vi "analise-motor.vi"() -> ()   [LabVIEW 2014]
panel:
  out "Waveform Graph":dbl[](graph)
  out "size(s)":i32
  out "subarray":dbl[](array[numeric]) format="%_20g"
  in  "Waveform Graph 2":dbl[][](graph)=[[0.0, 0.0, 1.0, 1.0, 1.0, 1.0, 1.0, 1.0, 1.0, 1.0, 1.0, 1.0, 1.0, 1.0, 1.0, 1.0, 1.0, 1.0, 1.0, 1.0, 1.0, 1.0, 1.0, 1.0, 1.0, 1.0, 1.0, 1.0, 1.0, 1.0, 1.0, 1.0, 1.0, 1.0, 1.0, 1.0, 1.0, 1.0, 1.0, 1.0, 1.0, 1.0, 1.0, 1.0, 1.0, 1.0, 1.0, 1.0, 1.0, 1.0, 1.0, 1.0, 1.0, 1.0, 1.0, 1.0, 1.0, 1.0, 1.0, 1.0, 1.0, 1.0, 1.0, 1.0, 1.0, 1.0, 1.0, 1.0, 1.0, 1.0, 1.0, 1.0, 1.0, 0.0, 0.0, 0.0, 0.0, 0.0, 0.0, 0.0, 0.0, 0.0, 0.0, 0.0, 0.0, 0.0, 0.0, 0.0, 0.0, 0.0, 0.0, 0.0, 0.0, 0.0, 0.0, 0.0, 0.0, 0.0, 0.0, 0.0, 0.0, 0.0, 0.0, 0.0, 0.0, 0.0, 0.0, 0.0, 0.0, 0.0], [0.0, 0.0, 0.0, 0.011164878731343308, 0.011164878731343308, 0.011164878731343308, 0.011164878731343308, 0.011164878731343308, 0.10415694962686572, 0.10415694962686572, 0.10415694962686572, 0.10415694962686572, 0.29133628731343275, 0.29133628731343275, 0.29133628731343275, 0.29133628731343275, 0.29133628731343275, 0.5729652518656717, 0.5729652518656717, 0.5729652518656717, 0.5729652518656717, 0.947440531716418, 0.947440531716418, 0.947440531716418, 0.947440531716418, 0.947440531716418, 1.4163654384328357, 1.4163654384328357, 1.4163654384328357, 1.4163654384328357, 1.4163654384328357, 1.9599755130597014, 1.9599755130597014, 1.9599755130597014, 1.9599755130597014, 1.9599755130597014, 2.5121560167910446, 2.5121560167910446, 2.5121560167910446, 2.5121560167910446, 3.0620044309701493, 3.0620044309701493, 3.0620044309701493, 3.0620044309701493, 3.0620044309701493, 3.604390158582089, 3.604390158582089, 3.604390158582089, 3.604390158582089, 3.604390158582089, 4.070195895522388, 4.070195895522388, 4.070195895522388, 4.070195895522388, 4.440794076492537, 4.440794076492537, 4.440794076492537, 4.440794076492537, 4.440794076492537, 4.717788013059701, 4.717788013059701, 4.717788013059701, 4.717788013059701, 4.717788013059701, 4.901294309701492, 4.901294309701492, 4.901294309701492, 4.901294309701492, 4.901294309701492, 4.99052588619403, 4.99052588619403, 4.99052588619403, 4.99052588619403, 5.000145755597015, 5.000145755597015, 5.000145755597015, 5.000145755597015, 5.000145755597015, 5.000029151119403, 5.000029151119403, 5.000029151119403, 5.000029151119403, 5.000029151119403, 5.0, 5.0, 5.0, 5.0, 5.0, 5.0, 5.0, 5.0, 5.0, 5.0, 5.0, 5.0, 5.0, 5.0, 5.0, 5.0, 5.0, 5.0, 5.0, 5.0, 5.0, 5.0, 5.0, 5.0, 5.0, 5.0, 5.0]]
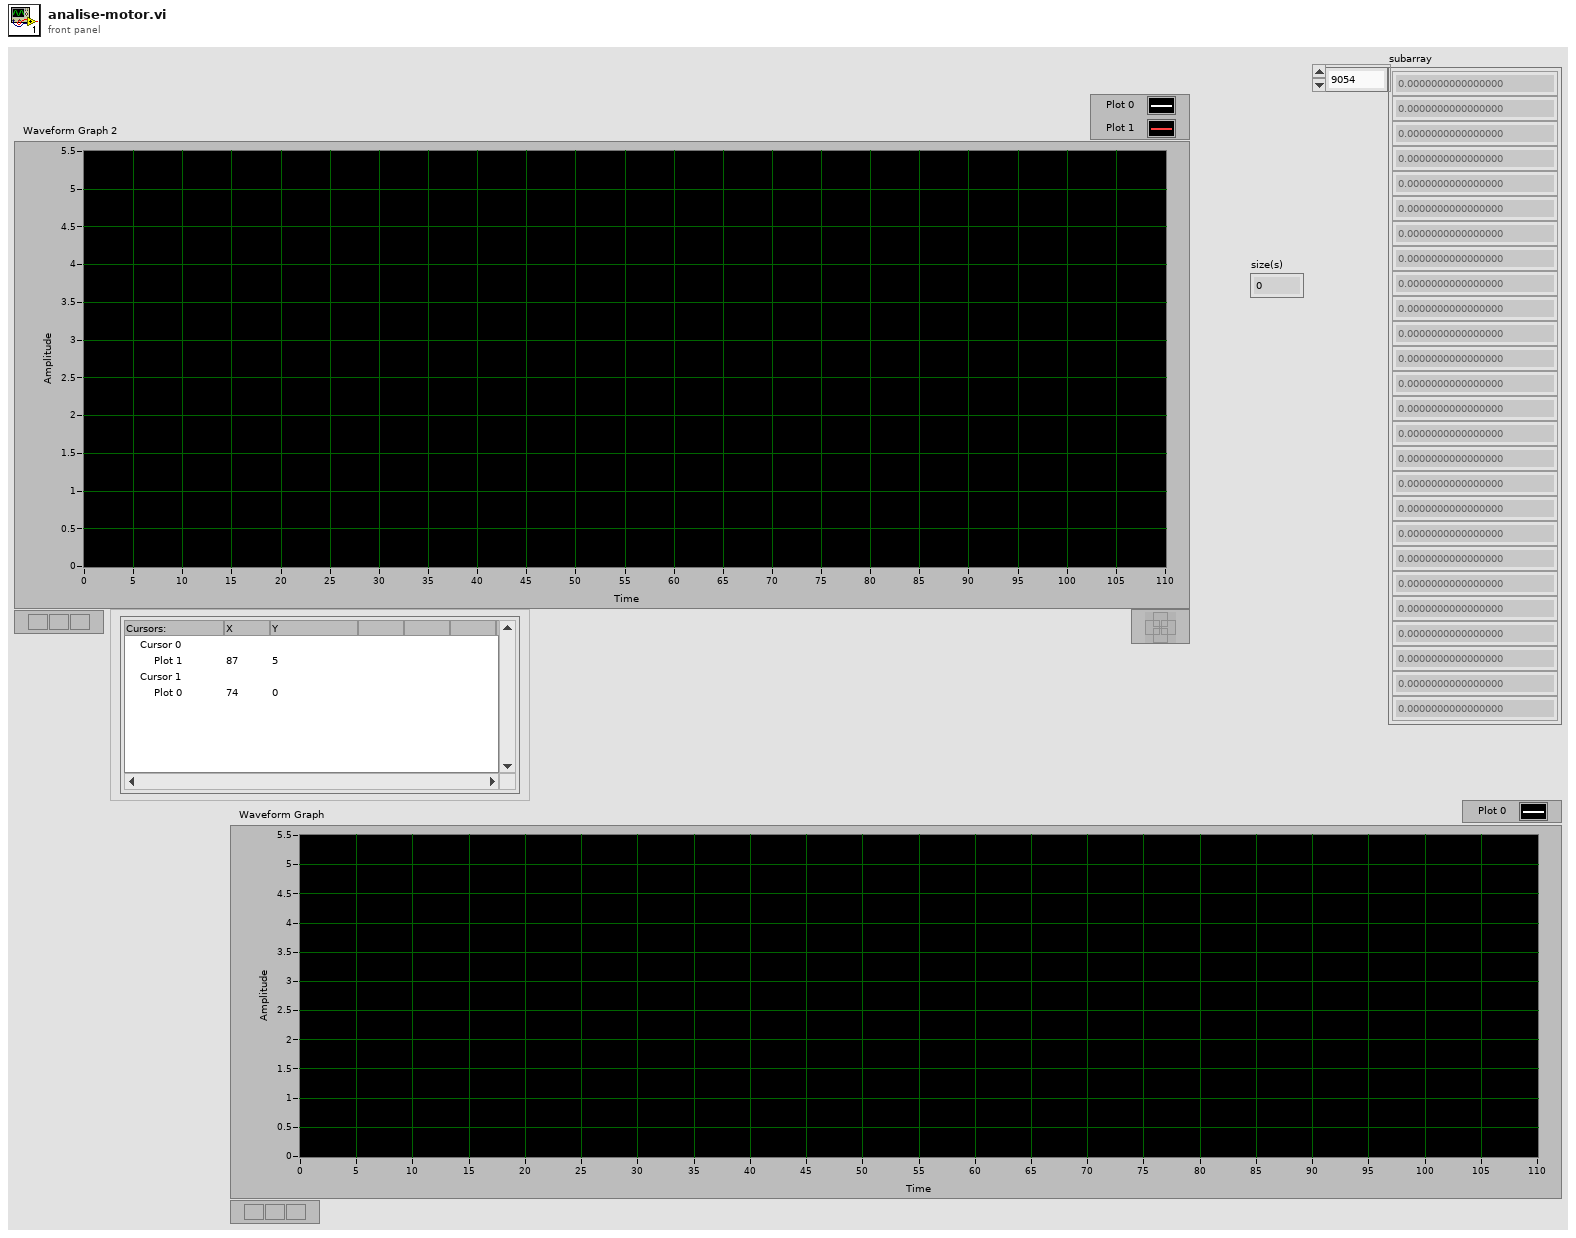
[diagram p1: front panel]
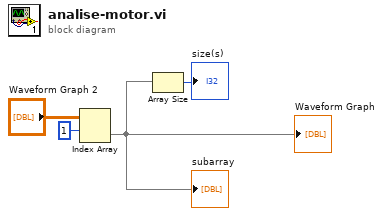
[diagram p0: block diagram]
diagram:
  n1 = Index Array(array="Waveform Graph 2", index (row)=1) -> (element=w1:dbl[])  [unwired: 1 in]
  "subarray" <- w1
  "Waveform Graph" <- w1
  n2 = Array Size(array=w1) -> (size(s)=→"size(s)":i32)
